vi "Day 4 - Camp Cleanup.vi"() -> ()   [LabVIEW 2020, in "AoC 2022.lvlib"]
uses:
  AoC 2022.lvlib
panel:
  out "Puzzle Part-2 Answer":string
  out "Puzzle Answer":string
  in  "Puzzle Input":string="2-4,6-8\n2-3,4-5\n5-7,7-9\n2-8,3-7\n6-6,4-6\n2-6,4-8"
  # "Enter the Puzzle Input and run the VI"
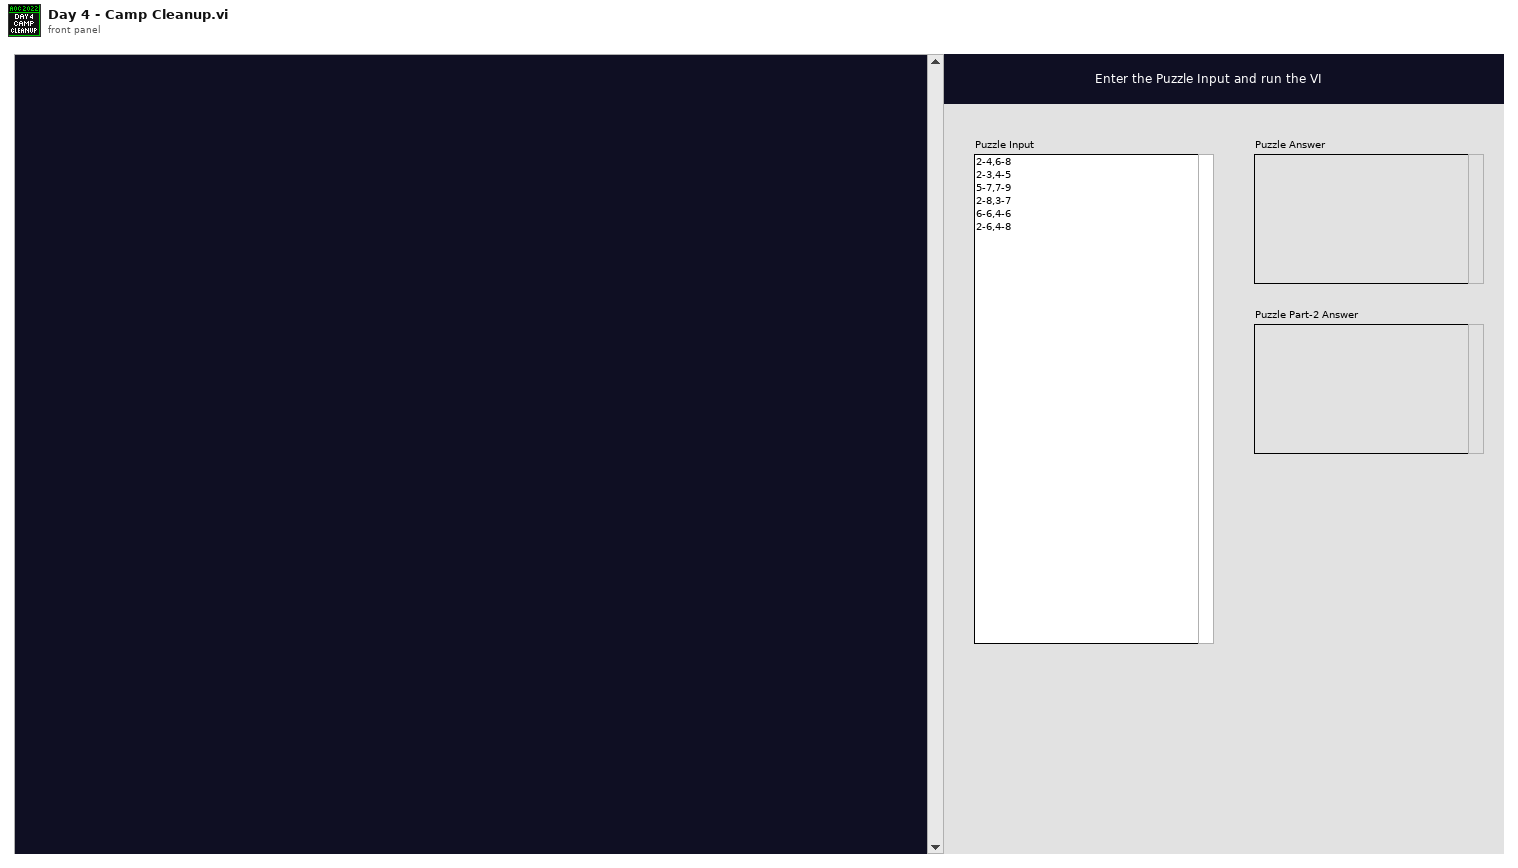
[diagram p1: front panel]
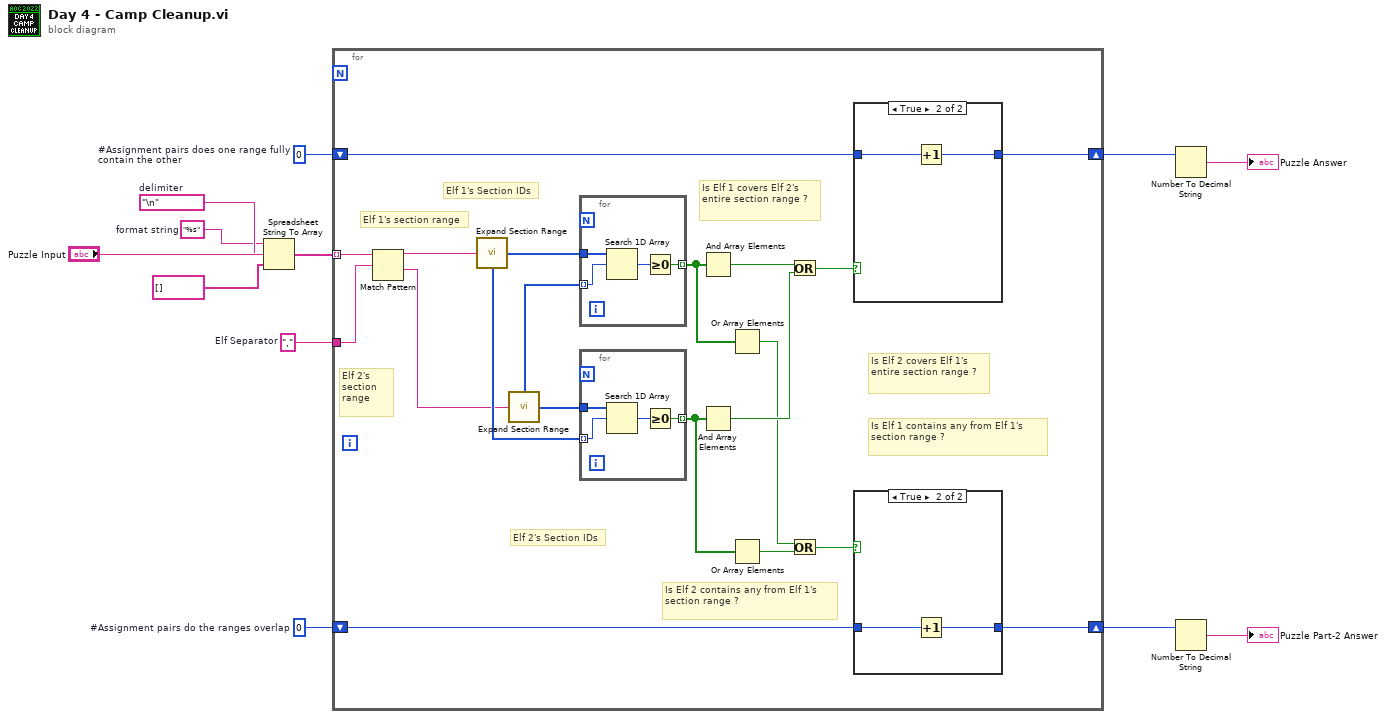
[diagram p0: block diagram]
diagram:
  w3 = 0  # #Assignment pairs do the ranges overlap
  w4 = 0  # #Assignment pairs does one range fully contain the other
  w5 = ","  # Elf Separator
  w10 = "%s"  # format string
  w11 = "\n"  # delimiter
  n1 = Spreadsheet String To Array(delimiter (Tab)=w11, format string=w10, spreadsheet string="Puzzle Input", array type (2D Dbl)=string[] []) -> (array=w6:string[])
  n2 = for {
    tunnel: w6 -> [w32] mode=indexing
    tunnel: w5 -> [w31]
    shift-right: [w21] -> w2
    shift-left: w4 -> [w22]
    shift-right: [w17] -> w1
    shift-left: w3 -> [w18]
    # "Is Elf 2 contains any from Elf 1's section range ?"
    # "Is Elf 1 contains any from Elf 1's section range ?"
    # "Is Elf 2 covers Elf 1's entire section range ?"
    # "Is Elf 1 covers Elf 2's entire section range ?"
    # "Elf 2's Section IDs"
    # "Elf 1's Section IDs"
    # "Elf 2's section range"
    # "Elf 1's section range"
    n3 = Match Pattern(string=w32, regular expression=w31) -> (before substring=w28:string, after substring=w20:string)  [unwired: 1 in, 2 out]
    n4 = call "Expand Section Range.vi"("Section Range"=w28) -> ("Section IDs"=w30:i32[], "Section End Points"=w26:i32[])  [unwired: 2 in]
    n5 = call "Expand Section Range.vi"("Section Range"=w20) -> ("Section IDs"=w29:i32[], "Section End Points"=w27:i32[])  [unwired: 2 in]
    n6 = for {
      tunnel: w30 -> [w46]
      tunnel: w27 -> [w45] mode=indexing
      tunnel: [w43] -> w16 mode=indexing
      n7 = Search 1D Array(1D array=w46, element=w45) -> (index of element=w44:i32)  [unwired: 1 in]
      n8 = Greater Or Equal To 0?(x=w44) -> (x >= 0?=w43:bool)
    }
    n9 = for {
      tunnel: w29 -> [w42]
      tunnel: w26 -> [w41] mode=indexing
      tunnel: [w39] -> w19 mode=indexing
      n10 = Search 1D Array(1D array=w42, element=w41) -> (index of element=w40:i32)  [unwired: 1 in]
      n11 = Greater Or Equal To 0?(x=w40) -> (x >= 0?=w39:bool)
    }
    n12 = And Array Elements(Boolean array=w16) -> (logical AND=w25:bool)
    n13 = And Array Elements(Boolean array=w19) -> (logical AND=w24:bool)
    n14 = Or Array Elements(Boolean array=w16) -> (logical OR=w14:bool)
    n15 = Or Array Elements(Boolean array=w19) -> (logical OR=w15:bool)
    n16 = Or(x=w25, y=w24) -> (x .or. y?=w23:bool)
    n17 = Or(x=w14, y=w15) -> (x .or. y?=w13:bool)
    n18 = case shown="True" w23 {
      tunnel: w22 -> [w36 w38]
      tunnel: [w36 w37] -> w21
      frame False {
      }
      frame True {
        n19 = Increment(x=w38) -> (x+1=w37:i32)
      }
    }
    n20 = case shown="True" w13 {
      tunnel: w18 -> [w33 w35]
      tunnel: [w33 w34] -> w17
      frame False {
      }
      frame True {
        n21 = Increment(x=w35) -> (x+1=w34:i32)
      }
    }
  }
  n22 = Number To Decimal String(number=w2) -> (decimal integer string=→"Puzzle Answer":string)  [unwired: 1 in]
  n23 = Number To Decimal String(number=w1) -> (decimal integer string=→"Puzzle Part-2 Answer":string)  [unwired: 1 in]
